vi "test4-MacroWithNonLocalSubMessages.vi"(8 "error in":errorcluster, 11 "TestCase in":refnum<class "testcase-CSMResponse.lvclass">) -> (0 "error out":errorcluster, 3 "TestCase out":refnum<class "testcase-CSMResponse.lvclass">)   [LabVIEW 2017, in "testcase-CSMResponse.lvclass"]
uses:
  testcase-CSMResponse.lvclass
  0c6454a9-3719-4e31-9ff6-45b39d38beb6.vi
  2437fcdf-222d-44ea-9250-34e015767128.vi
  src/user.lib/_NEVSTOP/Communicable State Machine(CSM)/AdvanceAPI/CSM - Get Module Attribute.vi
  <vilib>/addons/_JKI Toolkits/VI Tester/TestCase.llb/TestCase.lvclass
  src/user.lib/_NEVSTOP/Communicable State Machine(CSM)/Communicable State Machine.lvlib
  CSM/CSM-Testcase.lvlib
  C:/Program Files (x86)/National Instruments/LabVIEW 2017/vi.lib/addons/_JKI Toolkits/VI Tester/TestCase.llb/TestCase.lvclass
panel:
  out "Loopcount":i32
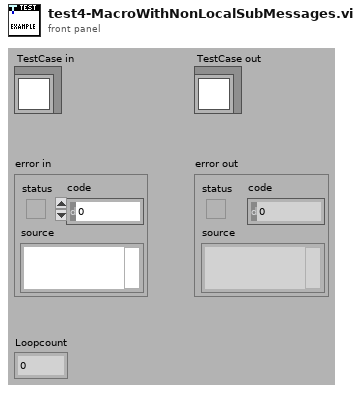
[diagram p1: front panel]
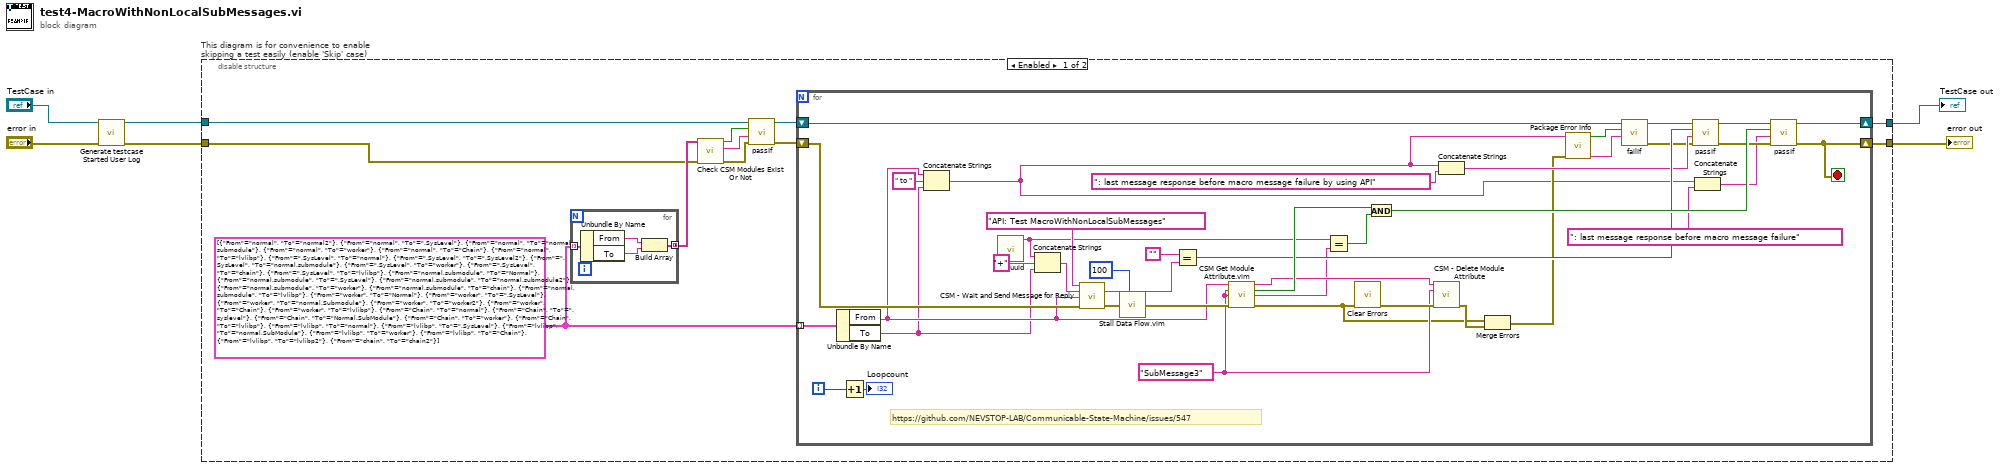
[diagram p0: block diagram]
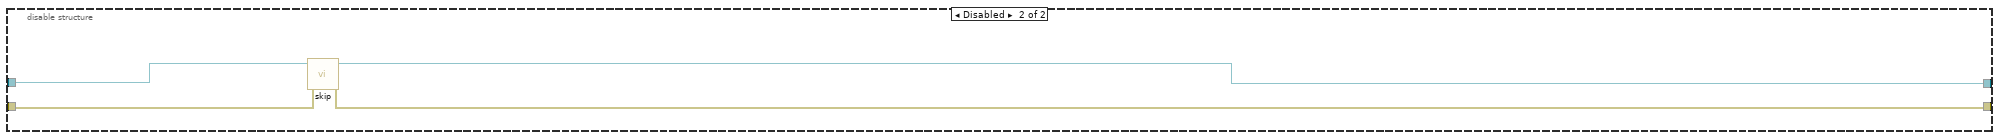
[diagram p2: hidden frame]
diagram:
  n1 = call "Generate testcase Started User Log.vi"("Error In"="error in") -> ("error out"=w1:errorcluster)  [unwired: 10 in]
  n2 = disable-structure "This diagram is for convenience to enable skipping a test easily (enable 'Skip' case)" shown="Enabled" {
    disable-tunnel: "TestCase in" -> [w7 w65]
    disable-tunnel: [w16 w63] -> w2
    disable-tunnel: [w15 w64] -> w4
    disable-tunnel: w1 -> [w9 w62]
    frame Enabled {
      w10 = cluster{"From":string, "To":string}[] [{"From"="normal", "To"="normal2"}, {"From"="normal", "To"=".SysLevel"}, {"From"="normal", "To"="normal.submodule"}, {"From"="normal", "To"="worker"}, {"From"="normal", "To"="Chain"}, {"From"="normal", "To"="lvlibp"}, {"From"=".SysLevel", "To"="normal"}, {"From"=".SysLevel", "To"=".SysLevel2"}, {"From"=".SysLevel", "To"="normal.submodule"}, {"From"=".SysLevel", "To"="worker"}, {"From"=".SysLevel", "To"="chain"}, {"From"=".SysLevel", "To"="lvlibp"}, {"From"="normal.submodule", "To"="Normal"}, {"From"="normal.submodule", "To"=".SysLevel"}, {"From"="normal.submodule", "To"="normal.submodule2"}, {"From"="normal.submodule", "To"="worker"}, {"From"="normal.submodule", "To"="chain"}, {"From"="normal.submodule", "To"="lvlibp"}, {"From"="worker", "To"="Normal"}, {"From"="worker", "To"=".SysLevel"}, {"From"="worker", "To"="normal.Submodule"}, {"From"="worker", "To"="worker2"}, {"From"="worker", "To"="Chain"}, {"From"="worker", "To"="lvlibp"}, {"From"="Chain", "To"="normal"}, {"From"="Chain", "To"=".syslevel"}, {"From"="Chain", "To"="Normal.SubModule"}, {"From"="Chain", "To"="worker"}, {"From"="Chain", "To"="lvlibp"}, {"From"="lvlibp", "To"="normal"}, {"From"="lvlibp", "To"=".SysLevel"}, {"From"="lvlibp", "To"="normal.SubModule"}, {"From"="lvlibp", "To"="worker"}, {"From"="lvlibp", "To"="Chain"}, {"From"="lvlibp", "To"="lvlibp2"}, {"From"="chain", "To"="chain2"}]
      n3 = for {
        tunnel: w10 -> [w20] mode=indexing
        tunnel: [w17] -> w13 mode=concatenating
        n4 = Unbundle By Name(w20) -> ("From"=w19:string, "To"=w18:string)
        n5 = Build Array(w19, w18) -> (w17:string[])
      }
      n6 = call "Check CSM Modules Exist Or Not.vi"("error in"=w9, "CSM names in"=w13) -> ("error out"=w11:errorcluster, "Debug string"=w12:string, "All Modules Exist?"=w14:bool)  [unwired: 7 in]
      n7 = call-dynamic "passIf.vi"("error in (no error)"=w11, "message (\"\")"=w12, "pass"=w14, "TestCase in"=w7) -> ("error out"=w8:errorcluster, "TestCase out"=w6:refnum<class "testcase-CSMResponse.lvclass">)  [unwired: 6 in]
      n8 = for {
        shift-right: [w49] -> w16
        shift-left: w6 -> [w25]
        shift-right: [w48] -> w15
        shift-left: w8 -> [w37]
        tunnel: w10 -> [w43] mode=indexing
        i -> [w61]
        stop <- w48 stop-if-true
        w50 = "SubMessage3" ("Attribute")
        # "https://github.com/NEVSTOP-LAB/Communicable-State-Machine/issues/547"
        n9 = Unbundle By Name(w43) -> ("From"=w33:string, "To"=w32:string)
        n10 = Increment(x=w61) -> (x+1=→"Loopcount":i32)
        n11 = Concatenate Strings(w33, " to " ("string"), w32) -> (w21:string)
        n12 = call "uuid.vi"() -> ("UUID"=w42:string)  [unwired: 11 in]
        n13 = Concatenate Strings(w42, "+", w32) -> (w40:string)
        n14 = call "CSM - Wait and Send Message for Reply.vi"("State"="API: Test MacroWithNonLocalSubMessages", "Arguments (\"\")"=w40, "Target Module"=w33, "Error In (No Error)"=w37) -> ("Response"=w47:string, "error out"=w59:errorcluster)  [unwired: 8 in, 2 out]
        n15 = call "Stall Data Flow.vim"("value in"=w59, "milliseconds to wait"=u32 100) -> ("value out"=w57:errorcluster)  [unwired: 1 out]
        n16 = Equal?(x="", y=w47) -> (x = y?=w46:bool)
        n17 = call "CSM Get Module Attribute.vim"("CSM Name"=w33, "Attribute"=w50, "Default Value (Empty Variant)"=w50, "Error In"=w57) -> ("CSM Name (Dup)"=w51:string, "Found"=w56:bool, "Value"=w39:string, "error out"=w35:errorcluster)  [unwired: 7 in, 1 out]
        n18 = Equal?(x=w42, y=w39) -> (x = y?=w54:bool)
        n19 = call <vilib>:"Clear Errors.vi"("error in (no error)"=w35) -> ("error out"=w52:errorcluster)  [unwired: 5 in, 1 out]
        n20 = And(x=w56, y=w54) -> (x .and. y?=w53:bool)
        n21 = call "CSM - Delete Module Attribute.vi"("CSM Name"=w51, "Attribute"=w50, "Error In"=w52) -> ("error out"=w36:errorcluster)  [unwired: 9 in, 3 out]
        n22 = Concatenate Strings(w21, ": last message response before macro message failure by using API" ("string")) -> (w30:string)
        n23 = Merge Errors(w35, w36) -> (w22:errorcluster)
        n24 = call "Package Error Info.vi"("error in"=w22, "String in"=w21) -> ("packed error info out"=w26:string, "error status"=w27:bool)  [unwired: 8 in]
        n25 = call-dynamic "failIf.vi"("message (\"\")"=w26, "fail"=w27, "TestCase in"=w25) -> ("error out"=w23:errorcluster, "TestCase out"=w24:refnum<class "testcase-CSMResponse.lvclass">)  [unwired: 7 in]
        n26 = call-dynamic "passIf.vi"("error in (no error)"=w23, "message (\"\")"=w30, "pass"=w46, "TestCase in"=w24) -> ("error out"=w44:errorcluster, "TestCase out"=w45:refnum<class "testcase-CSMResponse.lvclass">)  [unwired: 6 in]
        n27 = Concatenate Strings(w21, ": last message response before macro message failure" ("string")) -> (w28:string)
        n28 = call-dynamic "passIf.vi"("error in (no error)"=w44, "message (\"\")"=w28, "pass"=w53, "TestCase in"=w45) -> ("error out"=w48:errorcluster, "TestCase out"=w49:refnum<class "testcase-CSMResponse.lvclass">)  [unwired: 6 in]
      }
    }
    frame Disabled {
      # "skip test result while test is under development"
      n29 = call <vilib>:"skip.vi"("error in (no error)"=w62, "TestCase in"=w65) -> ("error out"=w64:errorcluster, "TestCase out"=w63:refnum<class "testcase-CSMResponse.lvclass">)  [unwired: 8 in]
    }
  }
  "error out" <- w4
  "TestCase out" <- w2
